vi "import_variables.vi"(11 "Module Search String":string="cDAQ1Mod1") -> (0 "Check Array":dbl[](array[numeric]), 3 "String Array From File":string[][](array[string]))   [LabVIEW 2017]
uses:
  <vilib>/Utility/file.llb/Read Delimited Spreadsheet (string).vi
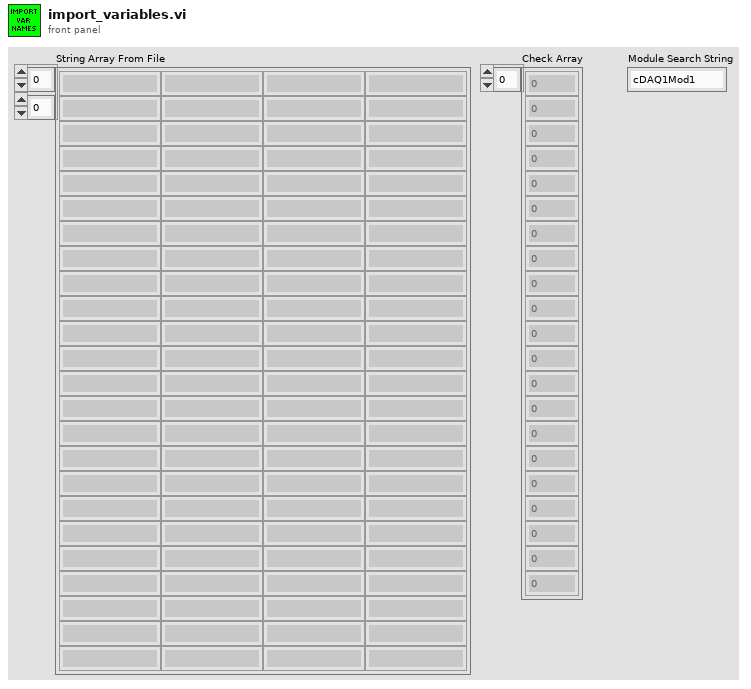
[diagram p1: front panel]
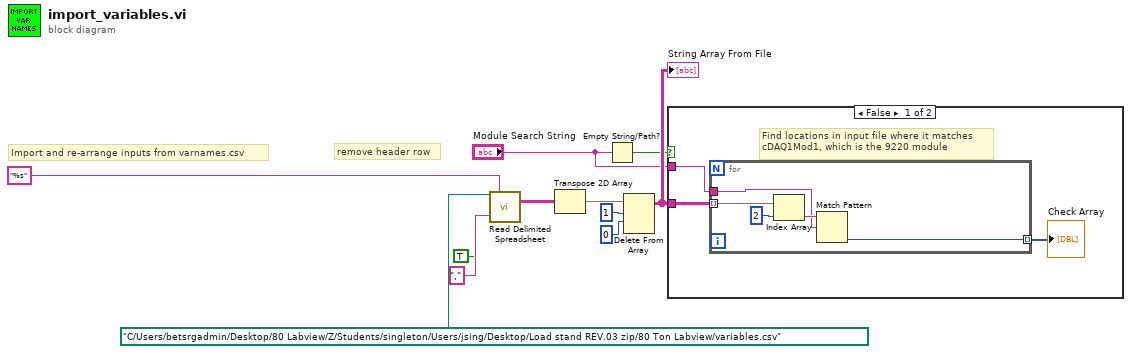
[diagram p0: block diagram]
diagram:
  # "remove header row"
  # "Import and re-arrange inputs from varnames.csv"
  n1 = call-poly <vilib>:"Read Delimited Spreadsheet.vi"("file path (dialog if empty)"=path "C:/Users/betsrgadmin/Desktop/80 Labview/Z/Students/singleton/Users/jsing/Desktop/Load stand REV.03 zip/80 Ton Labview/variables.csv", "format (%s)"="%s", "transpose? (F)"=TRUE, "delimiter (\\t)"=",") -> ("all rows"=w7:string[][])  [unwired: 6 in, 5 out]
  n2 = Transpose 2D Array(2D array=w7) -> (transposed array=w6:string[][])
  n3 = Empty String/Path?(string/path="Module Search String") -> (empty?=w2:bool)
  n4 = Delete From Array(array=w6, length=1, index (row)=0) -> (array with subset deleted=w3:string[][])  [unwired: 1 in, 1 out]
  "String Array From File" <- w3
  n5 = case shown="False" w2 {
    tunnel: w3 -> [w13 _]
    tunnel: "Module Search String" -> [w12 _]
    frame False {
      # "Find locations in input file where it matches\ncDAQ1Mod1, which is the 9220 module"
      n6 = for {
        tunnel: w13 -> [w19] mode=indexing
        tunnel: [w17] -> w14 mode=indexing
        tunnel: w12 -> [w15]
        n7 = Index Array(array=w19, index=2) -> (element=w18:string)
        n8 = Match Pattern(string=w18, regular expression=w15) -> (offset past match=w17:i32)  [unwired: 1 in, 3 out]
      }
      "Check Array" <- w14
    }
    frame True {
    }
  }
